vi "BundleToString.vi"(10 "Cluster":T1, 11 "String 2":string) -> (3 "String":string)   [LabVIEW 2017]
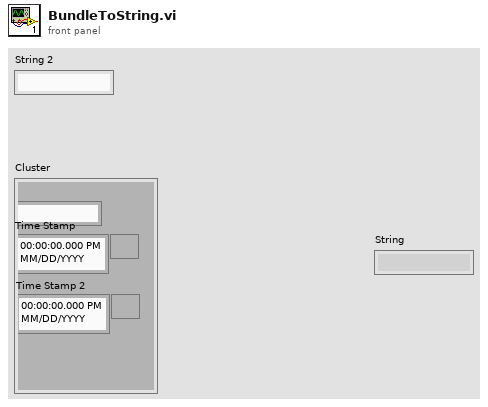
[diagram p1: front panel]
types:
  T1 = cluster{"String":string, "Time Stamp":timestamp, "Time Stamp 2":timestamp}
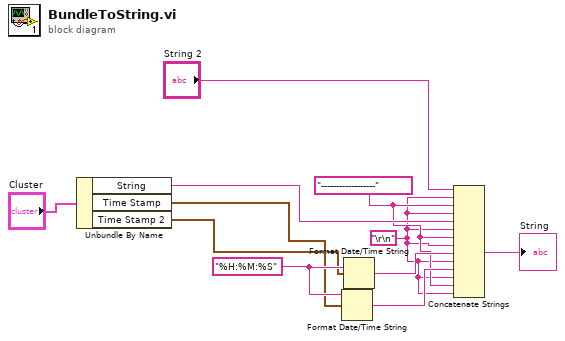
[diagram p0: block diagram]
diagram:
  w2 = "------------------"
  w1 = "\r\n"
  w9 = "%H:%M:%S"
  n1 = Unbundle By Name("Cluster") -> ("String"=w7:string, "Time Stamp"=w6:timestamp, "Time Stamp 2"=w5:timestamp)
  n2 = Format Date/Time String(time format string (%c)=w9, seconds (now)=w6) -> (date/time string=w11:string)  [unwired: 1 in]
  n3 = Format Date/Time String(time format string (%c)=w9, seconds (now)=w5) -> (date/time string=w10:string)  [unwired: 1 in]
  n4 = Concatenate Strings("String 2", w1, w2, w1, w7, w1, w2, w1, w10, w1, w11, w1, w2, w1) -> (→"String":string)
